vi "Add BDX to Tree.vi"(7 "AQT Name":string, 8 "error in (no error)":errorcluster, 9 "Path":path, 11 "TreeControl in":refnum<vi>) -> ()   [LabVIEW 2025]
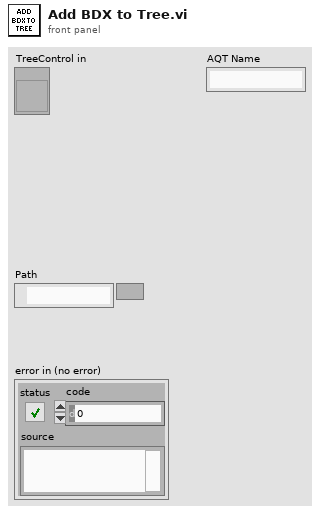
[diagram p1: front panel]
types:
  T1 = typedef "Decision Tree.ctl" = cluster{"Tree":T2[], "Node To Index Lookup Map":map{i16, i16[]}}
  T2 = typedef "Sequencing Tree Node.ctl" = cluster{"Node Type":enum16{"Path", "Command", "Leaf"}, "ID":i16, "Path Data":cluster{"Path Name":string, "Outcome Name":string}, "Single Cmd Info":T3, "Child ID":i32[], "Parent ID":i32, "Drawing Info":cluster{"X":i32, "Y":i32, "Width":i32, "Height":i32}}
  T3 = typedef "Single Cmd Info.ctl" = cluster{"Name":string, "CPTM.DataType":variant, "All Control Values Variant":cluster{"Name":string, "Variant Data":variant}[], "icon full":T4, "icon scaled":T4, "Path":path, "Subsystem Color":u32}
  T4 = typedef "imagedata.ctl" = cluster{"image type":i32, "image depth":i32, "image":u8[], "mask":u8[], "colors":u32[], "Rectangle":cluster{"left":i16, "top":i16, "right":i16, "bottom":i16}}
  T5 = cluster{"Path References":path[], "Decision Tree":T1}
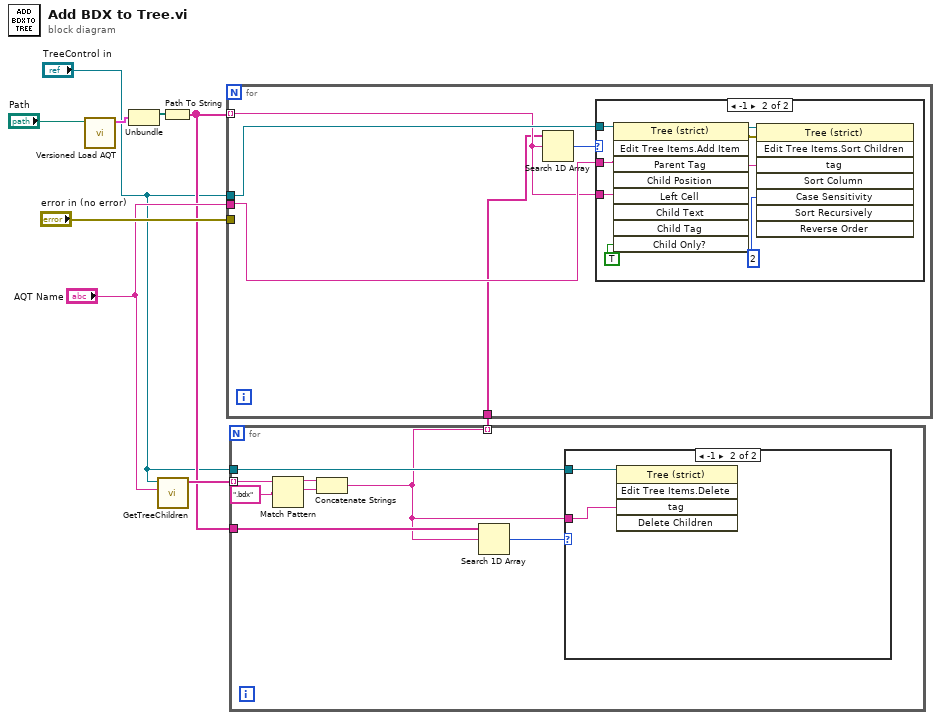
[diagram p0: block diagram]
diagram:
  n1 = call "Versioned Load AQT.vi"("Path"="Path") -> ("data"=w7:T5)  [unwired: 10 in]
  n2 = Unbundle(w7) -> ("Path References"=w6:path[])  [unwired: 1 out]
  n3 = call "GetTreeChildren.vi"("name"="AQT Name", "Tree 2"="TreeControl in") -> ("Children"=w5:string[])  [unwired: 9 in]
  n4 = Path To String(path=w6) -> (string=w2:string[])
  n5 = for {
    tunnel: w5 -> [w17] mode=indexing
    tunnel: [w10] -> w4 mode=indexing
    tunnel: w2 -> [w13]
    tunnel: "TreeControl in" -> [w11]
    n6 = Match Pattern(string=w17, regular expression=".bdx") -> (before substring=w15:string, match substring=w14:string)  [unwired: 1 in, 2 out]
    n7 = Concatenate Strings(w15, w14) -> (w10:string)
    n8 = Search 1D Array(1D array=w13, element=w10) -> (index of element=w12:i32)  [unwired: 1 in]
    n9 = case shown="-1" w12 {
      tunnel: w11 -> [_ w19]
      tunnel: w10 -> [_ w18]
      frame 0, Default {
      }
      frame -1 {
        n10 = invoke on="Invoke Node" class="Tree (strict)" method="Edit Tree Items.Delete"(reference=w19, "tag"=w18) -> ()  [unwired: 3 in, 5 out]
      }
    }
  }
  n11 = for {
    tunnel: w2 -> [w21] mode=indexing
    tunnel: "error in (no error)" -> [_]
    tunnel: "AQT Name" -> [w23]
    tunnel: "TreeControl in" -> [w22]
    tunnel: w4 -> [w20]
    n12 = Search 1D Array(1D array=w20, element=w21) -> (index of element=w24:i32)  [unwired: 1 in]
    n13 = case shown="-1" w24 {
      tunnel: w23 -> [_ w30]
      tunnel: w21 -> [_ w31]
      tunnel: w22 -> [_ w27]
      frame 0, Default {
      }
      frame -1 {
        n14 = invoke on="Invoke Node" class="Tree (strict)" method="Edit Tree Items.Add Item"(reference=w27, "Parent Tag"=w30, "Left Cell"=w31, "Child Only?"=TRUE) -> (reference out=w26:refnum<vi>, error out=w28:errorcluster)  [unwired: 5 in, 7 out]
        n15 = invoke on="Invoke Node" class="Tree (strict)" method="Edit Tree Items.Sort Children"(reference=w26, error in=w28, "tag"=w30, "Case Sensitivity"=2) -> ()  [unwired: 4 in, 8 out]
      }
    }
  }
